vi "tcp_monitor_get_dataList.vi"() -> ()   [LabVIEW 2021]
panel:
  out "data out 2":string[](array[string])
  out "value":T1(array[cluster])
  out "data out 3":string
  out "match substring":string[](array[string])
  in  "data out":string
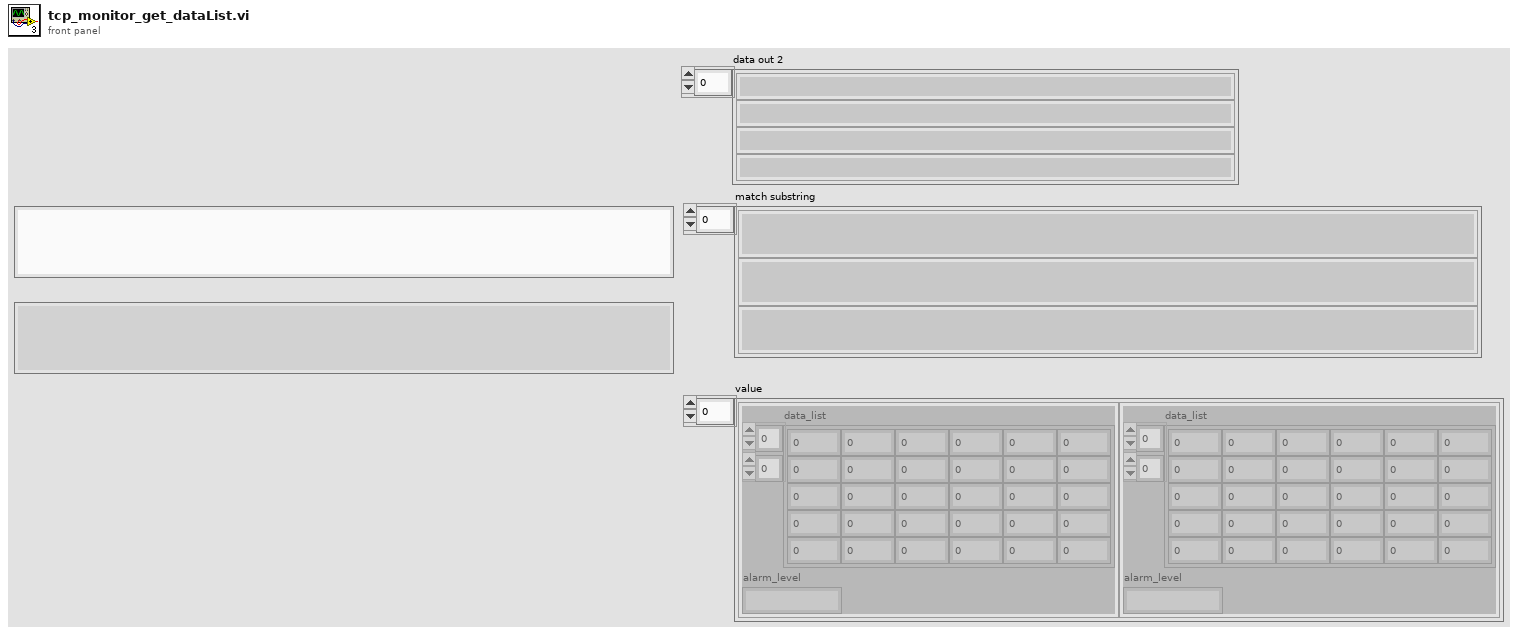
[diagram p1: front panel]
types:
  T1 = cluster{"data_list":dbl[][], "alarm_level":string}[]
  T2 = cluster{"data_list":dbl[][], "alarm_level":string}
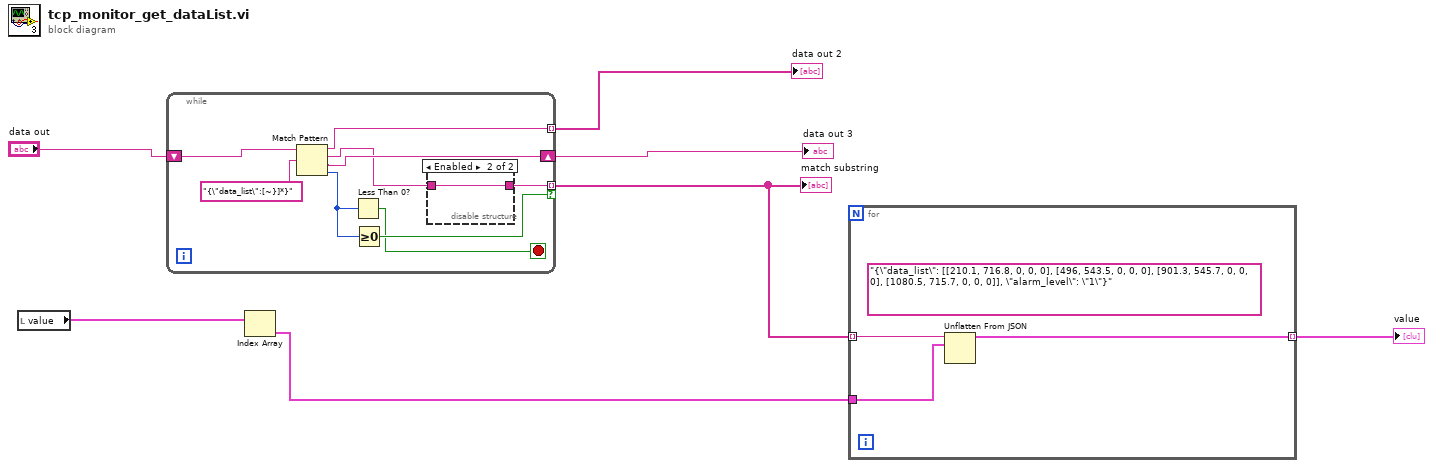
[diagram p0: block diagram]
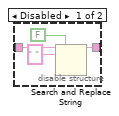
[diagram p2: hidden frame]
diagram:
  n1 = local read "value"() -> (w2:T1)
  n2 = while {
    shift-right: [w14] -> w6
    shift-left: "data out" -> [w16]
    tunnel: [w12] -> w5 mode=indexing if=w10
    tunnel: [w8] -> w4 mode=indexing
    stop <- w9 stop-if-true
    n3 = Match Pattern(string=w16, regular expression="{\"data_list\":[~}]*}") -> (before substring=w8:string, match substring=w13:string, after substring=w14:string, offset past match=w11:i32)  [unwired: 1 in]
    n4 = Less Than 0?(x=w11) -> (x < 0?=w9:bool)
    n5 = Greater Or Equal To 0?(x=w11) -> (x >= 0?=w10:bool)
    n6 = disable-structure shown="Enabled" {
      disable-tunnel: w13 -> [w20 w21]
      disable-tunnel: [w18 w21] -> w12
      frame Disabled {
        n7 = Search and Replace String(replace all?=FALSE ("replace all? (F)"), input string=w20, search string=" " ("substring (\"\")")) -> (result string=w18:string)  [unwired: 5 in, 3 out]
      }
      frame Enabled {
      }
    }
  }
  "match substring" <- w5
  "data out 3" <- w6
  "data out 2" <- w4
  n8 = Index Array(array=w2) -> (element=w1:T2)  [unwired: 1 in]
  n9 = for {
    tunnel: w5 -> [w24] mode=indexing
    tunnel: w1 -> [w23]
    tunnel: [w22] -> w3 mode=indexing
    (unwired) "{\"data_list\": [[210.1, 716.8, 0, 0, 0], [496, 543.5, 0, 0, 0], [901.3, 545.7, 0, 0, 0], [1080.5, 715.7, 0, 0, 0]], \"alarm_level\": \"1\"}" ("JSON string")
    n10 = Unflatten From JSON(JSON string=w24, type and defaults=w23) -> (value=w22:T2)  [unwired: 5 in, 1 out]
  }
  "value" <- w3
